vi "Station2_QR_Code_correct&localduplication_verification.vi"(9 "BARCODE STATION in":string, 10 "PART_NO":string, 11 "PRIVIOUS code":string[](array[string])) -> (2 "Correct part no True":bool, 3 "Correct part no & No duplication TRUE":bool)   [LabVIEW 2017]
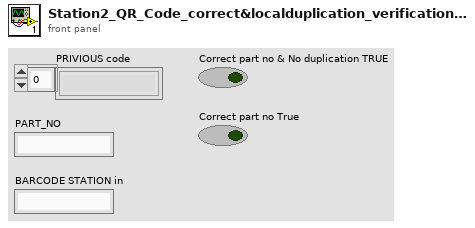
[diagram p1: front panel]
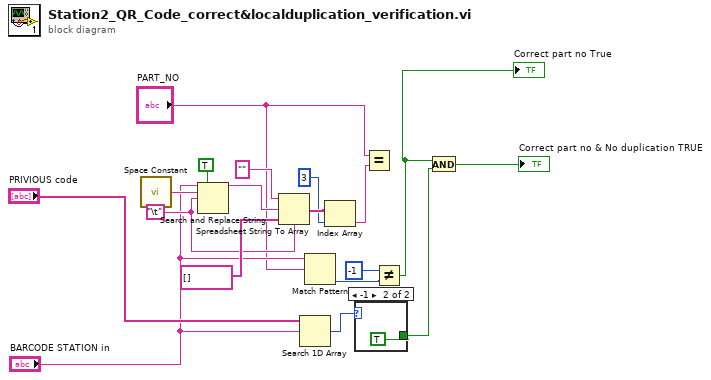
[diagram p0: block diagram]
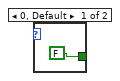
[diagram p2: hidden frame]
diagram:
  w9 = "\t"
  n1 = call <vilib>:"Space Constant.vi"() -> ("String"=w6:string)
  n2 = Search and Replace String(replace all?=TRUE ("replace all? (F)"), input string="BARCODE STATION in", search string=w6, replace string=w9) -> (result string=w8:string)  [unwired: 4 in, 3 out]
  n3 = Spreadsheet String To Array(delimiter (Tab)=w9, format string="", spreadsheet string=w8, array type (2D Dbl)=string[] []) -> (array=w13:string[])
  n4 = Search 1D Array(1D array="PRIVIOUS code", element="BARCODE STATION in") -> (index of element=w16:i32)  [unwired: 1 in]
  n5 = Match Pattern(string="BARCODE STATION in", regular expression="PART_NO") -> (offset past match=w3:i32)  [unwired: 1 in, 3 out]
  n6 = Index Array(array=w13, index=3) -> (element=w14:string)
  n7 = case shown="-1" w16 {
    tunnel: [FALSE TRUE] -> w17
    frame 0, Default {
    }
    frame -1 {
    }
  }
  n8 = Equal?(x="PART_NO", y=w14) -> ()  [unwired: 1 out]
  n9 = Not Equal?(x=-1, y=w3) -> (x != y?=w1:bool)
  "Correct part no True" <- w1
  n10 = And(x=w1, y=w17) -> (x .and. y?=→"Correct part no & No duplication TRUE":bool)
